vi "Some Base stuff.vi"(9 "Custom Shot Voltage":dbl, 10 "Custom Shot":bool, 11 "Shoot":bool) -> (3 "All Driver Commands":T1)   [LabVIEW 2012]
uses:
  All_Commands.ctl
  Climber/Climber_Commands.ctl
  Cirular Shooter/circular_shooter_commands.ctl
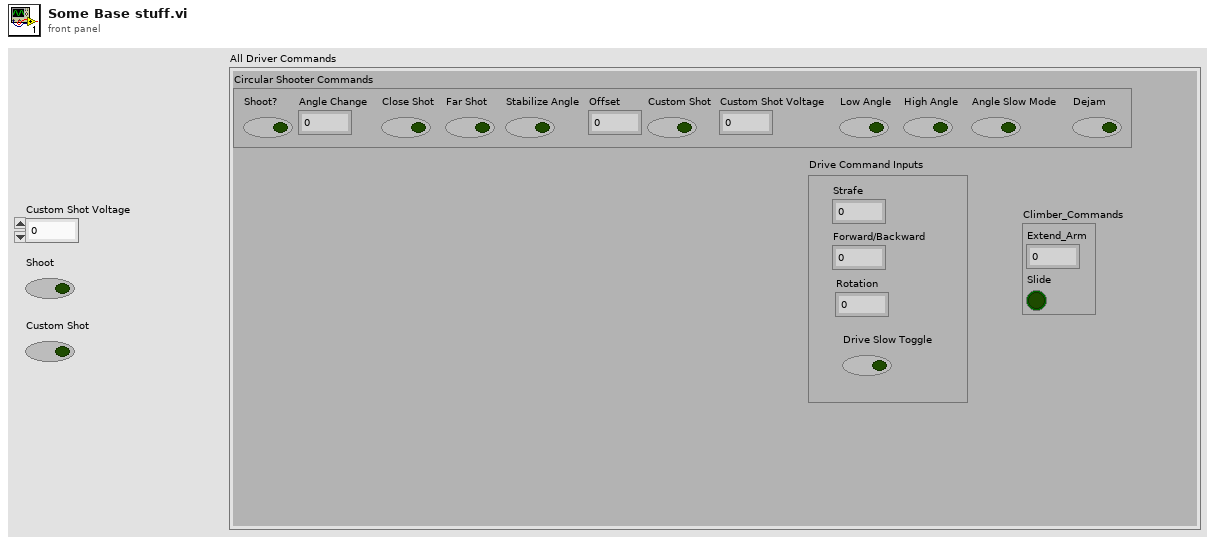
[diagram p1: front panel]
types:
  T1 = typedef "All_Commands.ctl" = cluster{"Circular Shooter Commands":T2, "Drive Command Inputs":cluster{"Strafe":dbl, "Forward/Backward":dbl, "Rotation":dbl, "Drive Slow Toggle":bool}, "Climber_Commands":T3}
  T2 = typedef "circular_shooter_commands.ctl" = cluster{"Shoot?":bool, "Angle Change":dbl, "Close Shot":bool, "Far Shot":bool, "Stabilize Angle ":bool, "Offset":dbl, "Custom Shot":bool, "Custom Shot Voltage":dbl, "Low Angle":bool, "High Angle":bool, "Angle Slow Mode":bool, "Dejam":bool}
  T3 = typedef "Climber_Commands.ctl" = cluster{"Extend_Arm":dbl, "Slide":bool}
  T4 = cluster{"Strafe":dbl, "Forward/Backward":dbl, "Rotation":dbl, "Drive Slow Toggle":bool}
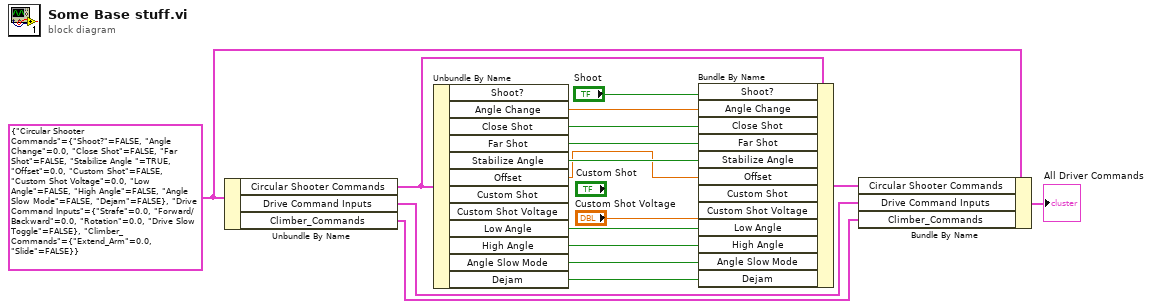
[diagram p0: block diagram]
diagram:
  w8 = T1 {"Circular Shooter Commands"={"Shoot?"=FALSE, "Angle Change"=0.0, "Close Shot"=FALSE, "Far Shot"=FALSE, "Stabilize Angle "=TRUE, "Offset"=0.0, "Custom Shot"=FALSE, "Custom Shot Voltage"=0.0, "Low Angle"=FALSE, "High Angle"=FALSE, "Angle Slow Mode"=FALSE, "Dejam"=FALSE}, "Drive Command Inputs"={"Strafe"=0.0, "Forward/Backward"=0.0, "Rotation"=0.0, "Drive Slow Toggle"=FALSE}, "Climber_Commands"={"Extend_Arm"=0.0, "Slide"=FALSE}} ("All Driver Commands")
  n1 = Unbundle By Name(w8) -> ("Circular Shooter Commands"=w17:T2, "Drive Command Inputs"=w6:T4, "Climber_Commands"=w5:T3)
  n2 = Unbundle By Name(w17) -> ("Angle Change"=w16:dbl, "Close Shot"=w15:bool, "Far Shot"=w14:bool, "Stabilize Angle"=w13:bool, "Offset"=w2:dbl, "Low Angle"=w12:bool, "High Angle"=w11:bool, "Angle Slow Mode"=w10:bool, "Dejam"=w9:bool)  [unwired: 3 out]
  n3 = Bundle By Name(cluster=w17, "Shoot?"="Shoot", "Angle Change"=w16, "Close Shot"=w15, "Far Shot"=w14, "Stabilize Angle"=w13, "Offset"=w2, "Custom Shot Voltage"="Custom Shot Voltage", "Low Angle"=w12, "High Angle"=w11, "Angle Slow Mode"=w10, "Dejam"=w9) -> (w7:T2)  [unwired: 1 in]
  n4 = Bundle By Name(cluster=w8, "Circular Shooter Commands"=w7, "Drive Command Inputs"=w6, "Climber_Commands"=w5) -> (→"All Driver Commands":T1)
